vi "BoxcarAverageBSPeed.vi"(2 "Boat Speed In":dbl, 3 "Box Car Average In":dbl[](array[numeric])) -> (0 "Boat Speed Out":dbl, 1 "Box Car Average Out":dbl[](array[numeric]))   [LabVIEW 2014]
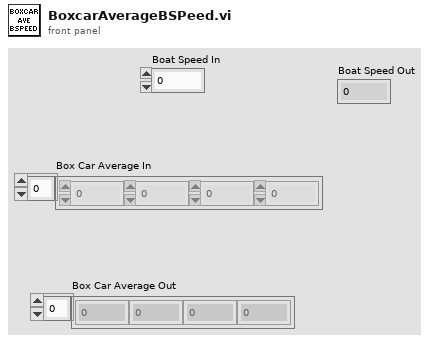
[diagram p1: front panel]
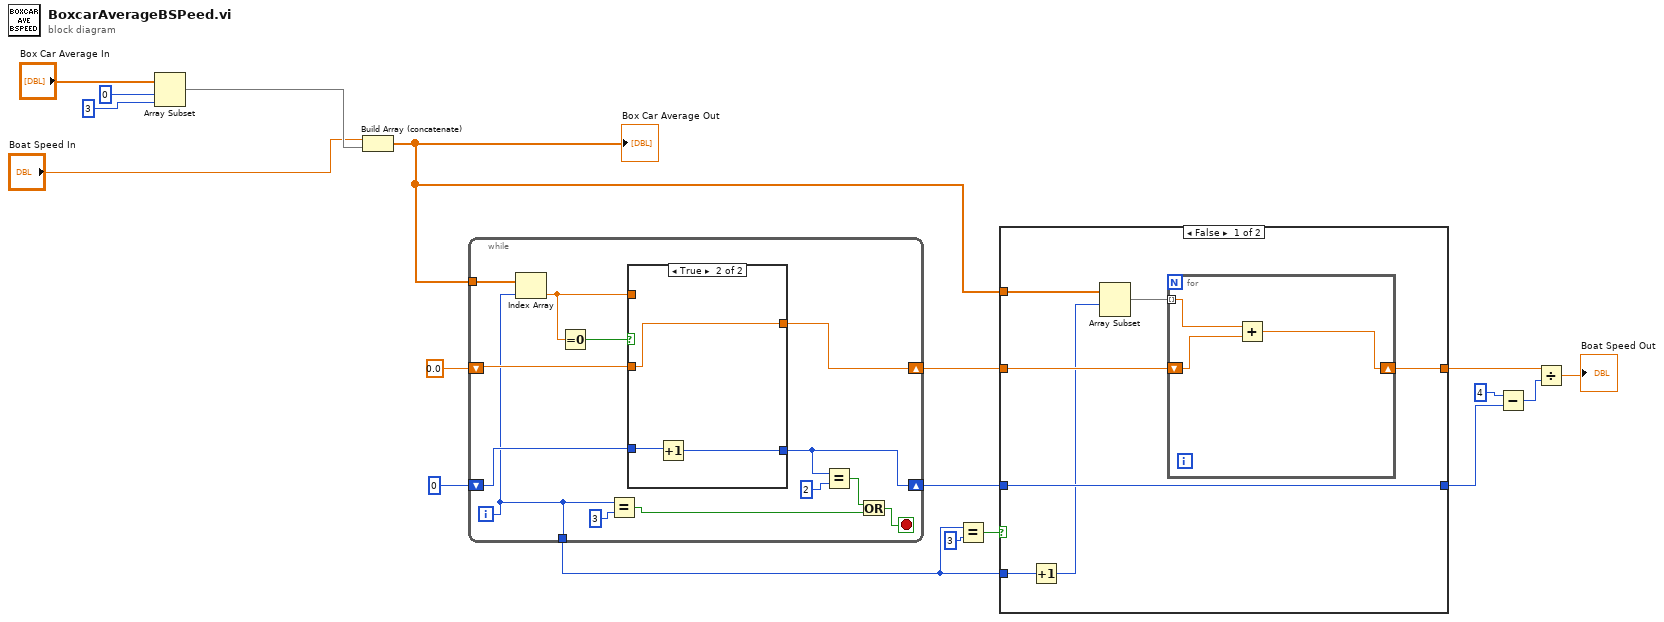
[diagram p0: block diagram]
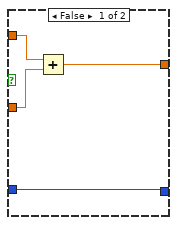
[diagram p3: hidden frame]
diagram:
  n1 = Array Subset(array="Box Car Average In", index=0, length=3) -> (w15:dbl[])
  n2 = Build Array (concatenate)("Boat Speed In", w15) -> (w11:dbl[])
  "Box Car Average Out" <- w11
  n3 = while {
    tunnel: w11 -> [w31]
    shift-right: [w27] -> w10
    shift-left: 0.0 -> [w28]
    shift-right: [w24] -> w5
    shift-left: 0 -> [w25]
    tunnel: [w19] -> w3
    i -> [w19]
    stop <- w22 stop-if-true
    n4 = Index Array "Index Array"(array=w31, index=w19) -> (element=w29:dbl)
    n5 = Equal To 0?(x=w29) -> (x = 0?=w30:bool)
    n6 = Equal?(x=w19, y=3) -> (x = y?=w20:bool)
    n7 = case shown="True" w30 {
      tunnel: w29 -> [w35 _]
      tunnel: w28 -> [w34 w36]
      tunnel: [w33 w36] -> w27
      tunnel: w25 -> [w32 w38]
      tunnel: [w32 w37] -> w24
      frame False {
        n8 = Add(x=w35, y=w34) -> (x+y=w33:dbl)
      }
      frame True {
        n9 = Increment(x=w38) -> (x+1=w37:i32)
      }
    }
    n10 = Equal?(x=w24, y=2) -> (x = y?=w21:bool)
    n11 = Or(x=w21, y=w20) -> (x .or. y?=w22:bool)
  }
  n12 = Equal?(x=w3, y=3) -> (x = y?=w1:bool)
  n13 = case shown="False" w1 {
    tunnel: w3 -> [w45 _]
    tunnel: w11 -> [w44 _]
    tunnel: w10 -> [w42 w50]
    tunnel: [w41 w50] -> w9
    tunnel: w5 -> [w40 w49]
    tunnel: [w40 w49] -> w4
    frame False {
      n14 = Increment(x=w45) -> (x+1=w39:i32)
      n15 = Array Subset "Array Subset"(array=w44, index=w39) -> (w43:dbl[])  [unwired: 1 in]
      n16 = for {
        tunnel: w43 -> [w48] mode=indexing
        shift-right: [w46] -> w41
        shift-left: w42 -> [w47]
        n17 = Add(x=w48, y=w47) -> (x+y=w46:dbl)
      }
    }
    frame True {
    }
  }
  n18 = Subtract(x=4, y=w4) -> (x-y=w8:i32)
  n19 = Divide(x=w9, y=w8) -> (x/y=→"Boat Speed Out":dbl)
